vi "Read Last CAN Configuration.vi"(8 "error in (no error)":errorcluster, 11 "Performanced XNET CAN Signal Logger in":refnum<class "Performanced XNET CAN Signal Logger.lvclass">) -> (0 "error out":errorcluster, 2 "Last CAN Configuration":refnum<data-value>, 3 "Performanced XNET CAN Signal Logger out":refnum<class "Performanced XNET CAN Signal Logger.lvclass">)   [LabVIEW 2021]
uses:
  Performanced XNET CAN Signal Logger.lvclass
  C:/Program Files/National Instruments/LabVIEW 2021/vi.lib/FlexLogger/SDK/PluginSDK.lvlibp/PEFClasses/SDK/Plugin/Plugin.lvclass
  C:/Program Files/National Instruments/LabVIEW 2021/vi.lib/FlexLogger/SDK/PluginSDK.lvlibp/PEFClasses/SDK/Processing Element/Processing Element.lvclass
  C:/Users/NI/Desktop/NIO DongZulong FlexLogger XNET/XNET-CAN-Signal-Logger/src/FlexLogger Plugin/Performanced XNET CAN Signal Logger.lvclass
  Typedef/Def-CAN Port Configuration.ctl
  XNET-CAN-Signal-Logger.lvlib
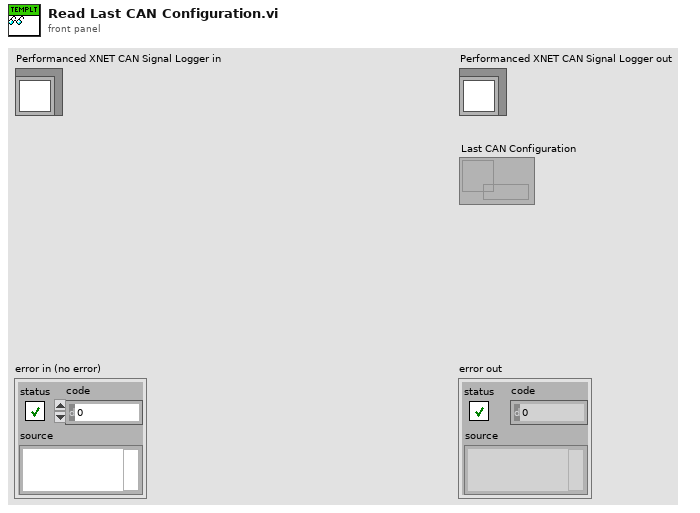
[diagram p1: front panel]
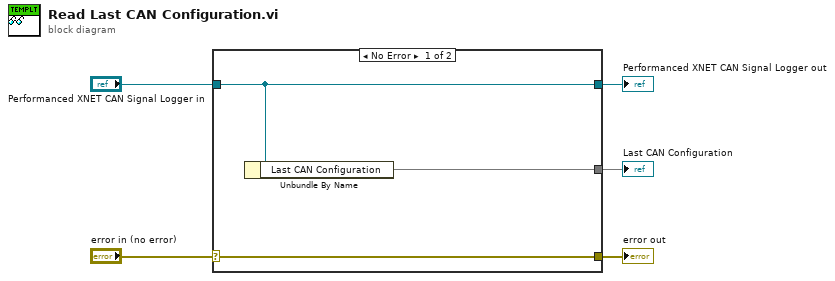
[diagram p0: block diagram]
diagram:
  n1 = case shown="No Error" "error in (no error)" {
    selector: "error in (no error)" -> [w8 w9]
    tunnel: [w8 w9] -> w4
    tunnel: [w7 w10] -> w2
    tunnel: "Performanced XNET CAN Signal Logger in" -> [w7 w10]
    tunnel: [w6 _] -> w1
    frame No Error {
      n2 = Unbundle By Name(w7) -> ("Last CAN Configuration"=w6)
    }
    frame Error {
    }
  }
  "error out" <- w4
  "Performanced XNET CAN Signal Logger out" <- w2
  "Last CAN Configuration" <- w1
